vi "Drawandpaint.vi"() -> ()   [LabVIEW 2021]
uses:
  <vilib>/Utility/miscctls.llb/LVPoint32TypeDef.ctl
  <vilib>/Instr/_visa.llb/VISA Configure Serial Port (Instr).vi
panel:
  in  "radius":i16=210
  in  "VISA resource name":refnum<visa-resource-name>
  in  "stop":bool
  out "2D Picture":picture
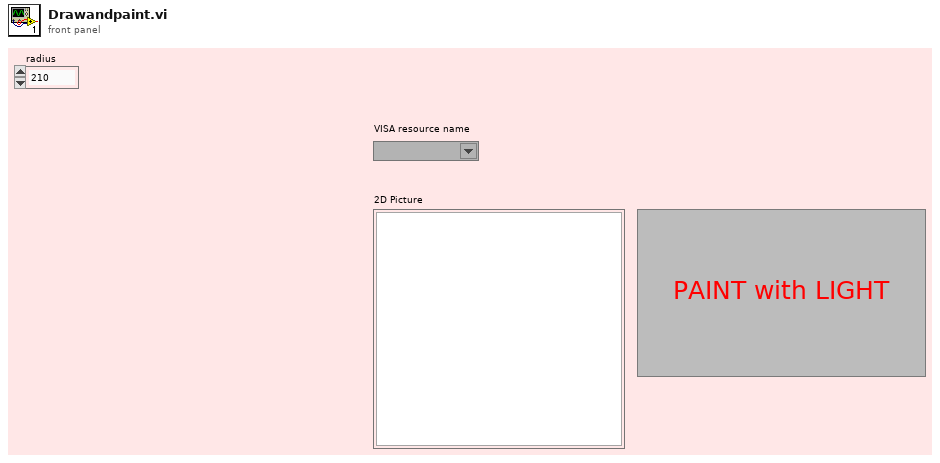
[diagram p1: front panel]
types:
  T1 = cluster{"left":i16, "top":i16, "right":i16, "bottom":i16}
  T2 = typedef "LVPoint32TypeDef.ctl" = cluster{"Horizontal":i32, "Vertical":i32}
  T3 = cluster{"Width":u16, "Style":enum32{"Solid", "Dash", "Dot", "DashDot", "DashDotDot"}}
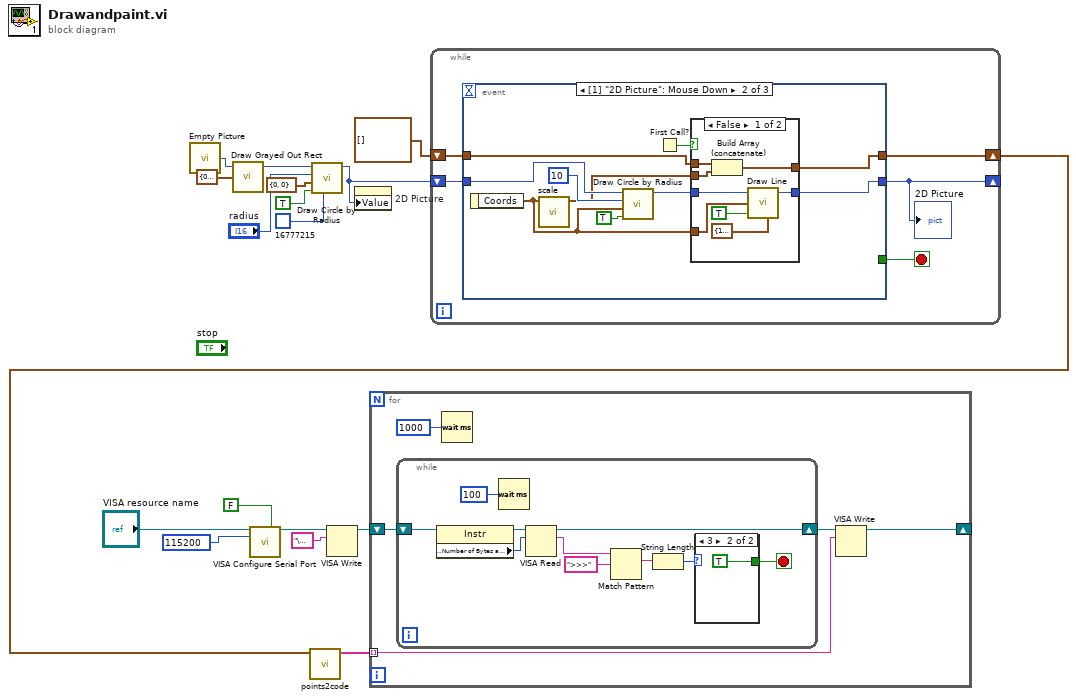
[diagram p0: block diagram]
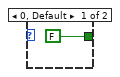
[diagram p2: hidden frame]
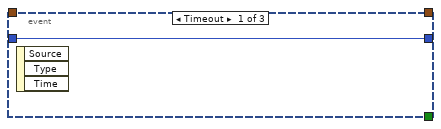
[diagram p3: hidden frame]
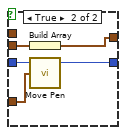
[diagram p4: hidden frame]
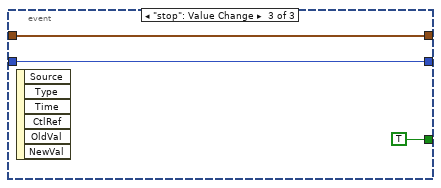
[diagram p5: hidden frame]
diagram:
  n1 = call "Empty Picture"() -> ("empty picture"=w12:picture)
  n2 = call <vilib>:"Draw Grayed Out Rect.vi"("rect"=T1 {"left"=0, "top"=0, "right"=500, "bottom"=500}, "picture"=w12) -> ("new picture"=w11:picture)  [unwired: 3 in]
  n3 = call-poly "VISA Configure Serial Port"("VISA resource name"="VISA resource name", "Enable Termination\nChar (T)"=FALSE ("Enable Termination\nChar (T)"), "baud rate (9600)"=u32 115200) -> ("VISA resource name out"=w1:refnum<visa-resource-name>)  [unwired: 11 in, 1 out]
  n4 = call <vilib>:"Draw Circle by Radius.vi"("color(black)"=u32 16777215, "fill?(F)"=TRUE, "pixel center"=cluster{"horizontal":i16, "vertical":i16} {"horizontal"=0, "vertical"=0}, "radius"="radius", "picture"=w11) -> ("new picture"=w9:picture)  [unwired: 6 in]
  n5 = VISA Write(VISA resource name=w1, write buffer="\u0004") -> (VISA resource name out=w3:refnum<visa-resource-name>)  [unwired: 1 in, 2 out]
  n6 = property on="2D Picture" class="Pict"("Value"=w9) -> ()  [unwired: 2 in, 2 out]
  n7 = while {
    shift-right: [w18] -> w2
    shift-left: T2[] [] -> [w21]
    shift-right: [w19] -> _
    shift-left: w9 -> [w20]
    stop <- w22 stop-if-true
    n8 = event shown="[1] \"2D Picture\": Mouse Down" {
      selector: _ -> [_ _ _]
      dyn-events: _ -> [_ _ _]
      timeout: _ -> [_ _ _]
      tunnel: [_ _ TRUE] -> w22
      tunnel: w21 -> [_ w31 w48]
      tunnel: [_ w32 w48] -> w18
      tunnel: w20 -> [w23 w30 w47]
      tunnel: [w23 w26 w47] -> w19
      event Timeout {
        n9 = event-data() -> ()  [unwired: 1 in, 3 out]
      }
      event "2D Picture": Mouse Down {
        n10 = event-data() -> ("Coords"=w25:T2)  [unwired: 1 in]
        n11 = call "scale.vi"("Coords in"=w25) -> ("Coords out"=w24:T2)  [unwired: 10 in]
        n12 = call <vilib>:"Draw Circle by Radius.vi"("fill?(F)"=TRUE, "pixel center"=w25, "radius"=i16 10, "picture"=w30) -> ("new picture"=w27:picture)  [unwired: 7 in]
        n13 = First Call?() -> (First Call?: T/F=w33:bool)
        n14 = case shown="False" w33 {
          tunnel: w24 -> [w35 w44]
          tunnel: [w40 w46] -> w32
          tunnel: w31 -> [w41 _]
          tunnel: w27 -> [w39 w45]
          tunnel: [w37 w43] -> w26
          tunnel: w25 -> [w34 w42]
          frame False {
            n15 = Build Array (concatenate)(w41, w35) -> (w40:T2[])
            n16 = call <vilib>:"Draw Line.vi"("picture"=w39, "end point"=w34, "absolute coordinates?(T)"=TRUE, "pen"=T3 {"Width"=10, "Style"=enum."Solid"}) -> ("new picture"=w37:picture)  [unwired: 5 in]
          }
          frame True {
            n17 = Build Array(w44) -> (w46:T2[])
            n18 = call <vilib>:"Move Pen.vi"("new position"=w42, "picture"=w45) -> ("new picture"=w43:picture)  [unwired: 3 in]
          }
        }
      }
      event "stop": Value Change {
        n19 = event-data() -> ()  [unwired: 1 in, 6 out]
      }
    }
    "2D Picture" <- w19
  }
  n20 = call "points2code.vi"("Array in"=w2) -> ("Array out"=w5:string[])  [unwired: 10 in]
  n21 = for {
    tunnel: w5 -> [w54] mode=indexing
    shift-right: [w52] -> _
    shift-left: w3 -> [w51]
    n22 = while {
      shift-right: [w60] -> w53
      shift-left: w51 -> [w55]
      stop <- w58 stop-if-true
      n23 = property class="Instr"(reference=w55) -> (reference out=w64:refnum<visa-resource-name>, "Serial Settings:Number of Bytes at Serial Port"=w63:u32)  [unwired: 1 in, 1 out]
      n24 = Wait (ms)(milliseconds to wait=u32 100) -> ()  [unwired: 1 out]
      n25 = VISA Read(VISA resource name=w64, byte count=w63) -> (VISA resource name out=w60:refnum<visa-resource-name>, read buffer=w57:string)  [unwired: 1 in, 2 out]
      n26 = Match Pattern(string=w57, regular expression=">>>") -> (match substring=w61:string)  [unwired: 1 in, 3 out]
      n27 = String Length(string=w61) -> (length=w59:i32)
      n28 = case shown="3" w59 {
        tunnel: [FALSE TRUE] -> w58
        frame 0, Default {
        }
        frame 3 {
        }
      }
    }
    n29 = Wait (ms)(milliseconds to wait=u32 1000) -> ()  [unwired: 1 out]
    n30 = VISA Write(VISA resource name=w53, write buffer=w54) -> (VISA resource name out=w52:refnum<visa-resource-name>)  [unwired: 1 in, 2 out]
  }
